vi "Run Action_Do.vi"(8 "error in (no error)":errorcluster, 10 "Project Builder in":refnum<class "Project Builder.lvclass">, 11 "PPL Class Test":refnum<class "PPL Class Test.lvclass">) -> (0 "error out":errorcluster, 1 "Success?":bool, 3 "Report":refnum<class "Report Data.lvclass">)   [LabVIEW 2020, in "ProjectBuilder.lvlib" / "PPL Class Test.lvclass"]
doc: "Run the action associated with the 'Project Action'-class.\n\nThis implementation load tests classes in PPL(s)."
uses:
  PPL Class Test.lvclass
  Data/Report Data/Report Data.lvclass
  Project Builder/Project Builder.lvclass
  PPL Class Test.lvclass/PPL Class Test.ctl
  PPL Class Test Data/PPL Class Test Data.lvclass/PPL Class Test Data.ctl
  PPL Class Test Data/PPL Class Test Data.lvclass
  C:/Current projects/WS/LV32.2020..ProjectBuilder/Class/Data/Report Data/Report Data.lvclass
  <vilib>/Utility/error.llb/Error Cluster From Error Code.vi
  <vilib>/ErrorRing/Error Ring.xnode
  ProjectBuilder.lvlib
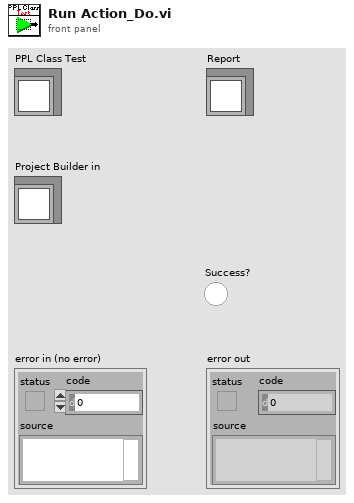
[diagram p1: front panel]
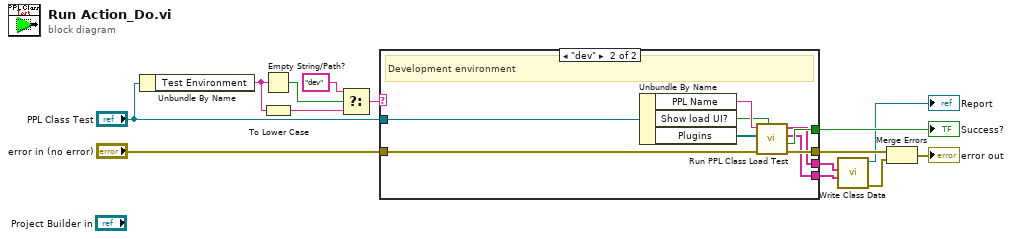
[diagram p0: block diagram]
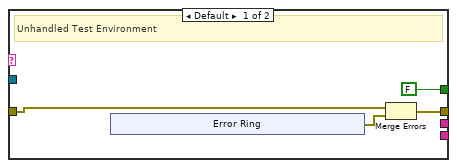
[diagram p2: hidden frame]
diagram:
  n1 = Unbundle By Name("PPL Class Test") -> ("Test Environment"=w13:string)
  n2 = Empty String/Path?(string/path=w13) -> (empty?=w14:bool)
  n3 = To Lower Case(string=w13) -> (all lower case string=w11:string)
  n4 = Select(t="dev", s=w14, f=w11) -> (s? t:f=w10:string)
  n5 = case shown="\"dev\"" w10 {
    tunnel: "error in (no error)" -> [w18 w29]
    tunnel: [w16 w28] -> w8
    tunnel: [FALSE w27] -> w7
    tunnel: "PPL Class Test" -> [_ w31]
    tunnel: [_ w26] -> w3
    tunnel: [_ w25] -> w2
    frame Default {
      # "Unhandled Test Environment"
      n6 = xnode "Error Ring"() -> ("error out"=w15:errorcluster)
      n7 = Merge Errors(w18, w15) -> (w16:errorcluster)
    }
    frame "dev" {
      # "Development environment"
      n8 = Unbundle By Name(w31) -> ("PPL Name"=w30:string, "Show load UI?"=w24:bool, "Plugins"=w23:refnum<class "PPL Class Test Plugin.lvclass">[])
      n9 = call "Run PPL Class Load Test.vi"("Show UI on Class load?(T)"=w24, "error in"=w29, "PPL Class Test Plugins"=w23, "PPL Name in PPL folder (entire PPL folder if empty)"=w30) -> ("error out"=w28:errorcluster, "Success?"=w27:bool, "Load Failure"=w25:string[], "Load Success"=w26:string[])  [unwired: 4 in]
    }
  }
  "Success?" <- w7
  n10 = call "Write Class Data.vi"("Load Failure"=w2, "Load Success"=w3) -> ("error out"=w4:errorcluster, "PPL Class Test Data out"=→"Report":refnum<class "PPL Class Test Data.lvclass">)  [unwired: 8 in]
  n11 = Merge Errors(w8, w4) -> (→"error out":errorcluster)
